vi "Window-Enter live trig width 26_01_18.vi"(8 "error in (no error)":errorcluster) -> (0 "error out":errorcluster)   [LabVIEW 2017]
doc: "Use this template to create a dialog box with event handling."
uses:
  <vilib>/Utility/miscctls.llb/LVPointTypeDef.ctl
  Global Variables/gl_UI Ctrl Refs.vi
  Global Variables/General Globals.vi
  Global Variables/FPGAstatus_Reference.vi
panel:
  in  "Pulse Width":dbl=0.1 min=0.1 max=0.9 step=0.1 format="%#.1f ms"
  in  "OK":bool
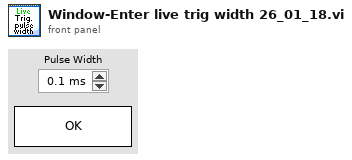
[diagram p1: front panel]
types:
  T1 = typedef "LVPointTypeDef.ctl" = cluster{"Horizontal":i16, "Vertical":i16}
  T2 = typedef "UI ctrl refs cluster.ctl" = cluster{"Top level VI path":path, "Top level VI ref":refnum<vi>, "User menu ref":refnum<k9>, "Sub Panel control":refnum<vi>, "Imaging Param Tab":T3, "Occurrence-Start drivers":refnum<k4>, "Occurrence-Speed logging initialised":refnum<k4>, "Occurrence-XYZ stage initialised":refnum<k4>, "Exit button":refnum<vi>, "Status ind":refnum<vi>, "Set as origin":refnum<vi>, "Speed Logging":refnum<vi>, "Time Lapse":refnum<vi>, "Live Imaging":refnum<vi>, "AOL Z Stack":refnum<vi>, "Motor Z Stack":refnum<vi>, "Funct Acq button":refnum<vi>, "Hard Shutter":refnum<vi>, "Virtual Shutter":refnum<vi>, "Laser Power":refnum<vi>, "AOL Mode":refnum<vi>, "Frame Size":refnum<vi>, "Field of View":refnum<vi>, "Dwell Time":refnum<vi>, "Zoom":refnum<vi>, "AOL Z":refnum<vi>, "Objective":refnum<vi>, "Axis":refnum<vi>, "Paths & Names":refnum<vi>, "Experiment folder path (ind.)":refnum<vi>, "Last State (Ind.)":refnum<vi>, "Laser wavelength ind (nm)":refnum<vi>, "Averages":refnum<vi>, "Angle (degrees)":refnum<vi>, "X centre":refnum<vi>, "Y centre":refnum<vi>, "Plane Mode":refnum<vi>, "# Planes":refnum<vi>, "Z Start":refnum<vi>, "Z Stop":refnum<vi>, "Z Step":refnum<vi>, "PMT 1":refnum<vi>, "PMT 2":refnum<vi>, "Stage XYZ Position":refnum<vi>, "Pockels@Z Start":refnum<vi>, "Pockels@Z Stop":refnum<vi>, "Obtain Z Start":refnum<vi>, "Obtain Z Stop":refnum<vi>, "Live stim.trig.period":refnum<vi>, "Live stim.trig.enable":refnum<vi>, "Movement Correction":refnum<vi>, "Load Reference Image":refnum<vi>, "XY Stage Move":refnum<vi>, "MovCor Cluster":refnum<vi>, "RefDAQParam":refnum<vi>, "Funct. Acq. Pockels Modulation":refnum<vi>, "Background MovCor":refnum<vi>, "Ref Laser Power":refnum<vi>, "Enable Video Recording":refnum<vi>, "Video Record-Live Imaging":refnum<vi>, "Video Record-Funct acq":refnum<vi>, "Reference Source":refnum<vi>, "AOL Z-stack Chirps Ready (ind)":refnum<vi>, "Target time between mov.cor. ref triggers (ms)":refnum<vi>, "Funct. Acq. Ref frame save":refnum<vi>, "Tracking button":refnum<vi>, "Show ref plots window":refnum<vi>, "Center freq ind (nm)":refnum<vi>, "Pickup mode (ind)":refnum<vi>, "Logging queue (ind)":refnum<vi>, "Back aperture power (ind.)":refnum<vi>, "Power after objective (ind.)":refnum<vi>, "Switch user":refnum<vi>, "Ls1 Conn. Status":refnum<vi>, "Ls1Tuning Status":refnum<vi>, "Ls1 Faults":refnum<vi>, "Ls1 Connection":refnum<vi>, "Ls1 Mode":refnum<vi>, "Ls1 POWER [mW]":refnum<vi>, "Ls1Shutter":refnum<vi>, "Ls1 Wavelength":refnum<vi>, "Ls1 message":refnum<vi>, "Ls1 Note":refnum<vi>, "Confirm Wav":refnum<vi>, "Ls1 PreChrp Prism1":refnum<vi>, "Ls1 PreChrp Prism2":refnum<vi>, "Laser Status Ind":refnum<vi>}
  T3 = typedef "Imaging Param ref.ctl" = refnum<vi>
  T4 = typedef "FPGA Ref.ctl" = refnum<k20>
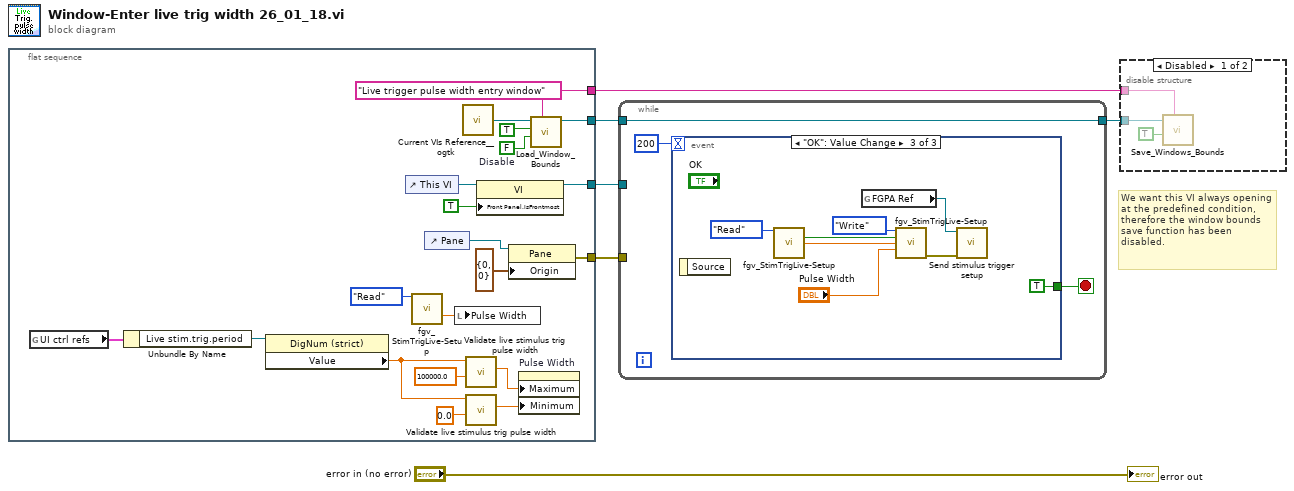
[diagram p0: block diagram]
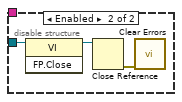
[diagram p2: hidden frame]
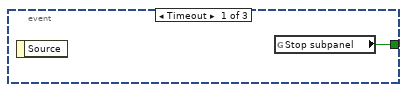
[diagram p3: hidden frame]
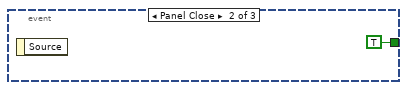
[diagram p4: hidden frame]
diagram:
  # "We want this VI always opening at the predefined condition, therefore the window bounds save function has been disabled."
  n1 = flat-sequence {
    tunnel: [w24] -> w6
    tunnel: [w22] -> w5
    tunnel: [w18] -> w4
    tunnel: [w17] -> w3
    frame #0 {
      w19 = FALSE  # Disable
      w18 = "Live trigger pulse width entry window" ("Window Name (i.e. Key)")
      n2 = global read "gl_UI Ctrl Refs.vi" "UI ctrl refs"() -> (w11:T2)
      n3 = Unbundle By Name(w11) -> ("Live stim.trig.period"=w10:refnum<vi>)
      n4 = property class="DigNum (strict)"(reference=w10) -> ("Value"=w9:dbl)  [unwired: 1 in, 2 out]
      n5 = control-ref of="This VI"() -> (w25:refnum<vi>)
      n6 = call "fgv_StimTrigLive-Setup.vi"("Function"=enum16{"Intialize", "Write", "Read", "Clear"}."Read") -> ("Live stim.trig.width (ms)"=w15:dbl)  [unwired: 11 in, 3 out]
      n7 = control-ref of="Pane"() -> (w21:refnum<vi>)
      n8 = local write "Pulse Width"(w15) -> ()
      n9 = call <userlib>:"Current VIs Reference__ogtk.vi"() -> ("Current VI's reference"=w20:refnum<vi>)  [unwired: 5 in]
      n10 = call "Validate live stimulus trig pulse width.vi"("Requested trigger pulse width (ms)"=100000.0, "Trigger period (sec)"=w9) -> ("Live imaging. stimulus trigger pulse width (ms)"=w8:dbl)  [unwired: 9 in]
      n11 = call "Validate live stimulus trig pulse width.vi"("Requested trigger pulse width (ms)"=0.0, "Trigger period (sec)"=w9) -> ("Live imaging. stimulus trigger pulse width (ms)"=w7:dbl)  [unwired: 9 in]
      n12 = property on="Property Node" class="VI"(reference=w25, "Front Panel.IsFrontmost"=TRUE ("Front Panel Window:Is Frontmost")) -> (reference out=w24:refnum<vi>)  [unwired: 1 in, 1 out]
      n13 = property class="Pane"(reference=w21, "Origin"=T1 {"Horizontal"=0, "Vertical"=0}) -> (error out=w22:errorcluster)  [unwired: 1 in, 1 out]
      n14 = property on="Pulse Width" class="DigNum (strict)"("Maximum"=w8, "Minimum"=w7) -> ()  [unwired: 2 in, 2 out]
      n15 = call "Load_Window_Bounds.vi"("Window Name (i.e. Key)"=w18, "Disable"=w19, "First Call"=TRUE, "Window VI's Ref"=w20) -> ("reference out"=w17:refnum<vi>)  [unwired: 4 in, 3 out]
    }
  }
  n16 = while {
    tunnel: w5 -> [_]
    tunnel: w6 -> [_]
    tunnel: w3 -> [w27]
    tunnel: [w27] -> w2
    stop <- w29 stop-if-true
    n17 = event shown="[2] \"OK\": Value Change" {
      selector: _ -> [_ _ _]
      dyn-events: _ -> [_ _ _]
      timeout: 200 -> [_ _ _]
      tunnel: [w30 TRUE ("Stop?") TRUE ("Stop?")] -> w29
      event Timeout {
        n18 = event-data() -> ()  [unwired: 1 in, 1 out]
        n19 = global read "General Globals.vi" "Stop subpanel"() -> (w30:bool)
      }
      event Panel Close {
        n20 = event-data() -> ()  [unwired: 1 in, 1 out]
      }
      event "OK": Value Change {
        n21 = event-data() -> ()  [unwired: 1 in, 1 out]
        n22 = call "fgv_StimTrigLive-Setup.vi"("Function"=enum16{"Intialize", "Write", "Read", "Clear"}."Read") -> ("Live stim.trig.enable"=w36:bool, "Live stim.trig.period (sec)"=w35:dbl)  [unwired: 11 in, 2 out]
        n23 = global read "FPGAstatus_Reference.vi" "FGPA Ref"() -> (w34:T4)
        n24 = call "fgv_StimTrigLive-Setup.vi"("Function"=enum16{"Intialize", "Write", "Read", "Clear"}."Write", "Live stim.trig.enable"=w36, "Live stim.trig.period (sec)"=w35, "Live stim.trig.width (ms)"="Pulse Width") -> ("error out"=w33:errorcluster)  [unwired: 8 in, 3 out]
        n25 = call "Send stimulus trigger setup.vi"("error in (no error)"=w33, "FPGA ref in"=w34) -> ()  [unwired: 8 in, 2 out]
      }
    }
  }
  n26 = disable-structure shown="Disabled" {
    disable-tunnel: w4 -> [w42 _]
    disable-tunnel: w2 -> [w40 w43]
    frame Disabled {
      n27 = call "Save_Windows_Bounds.vi"("Window Name (i.e. Key)"=w42, "Front Panel Window:Open"=TRUE, "Window VI's Ref"=w40) -> ()  [unwired: 8 in, 1 out]
    }
    frame Enabled {
      n28 = invoke class="VI" method="FP.Close"(reference=w43) -> (reference out=w44:refnum<vi>)  [unwired: 2 in, 2 out]
      n29 = Close Reference(reference=w44) -> (error out=w45:errorcluster)  [unwired: 1 in]
      n30 = call <vilib>:"Clear Errors.vi"("error in (no error)"=w45) -> ()  [unwired: 5 in, 2 out]
    }
  }
  "error out" <- "error in (no error)"
